vi "Spam - Wait.vi"(8 "Error In":errorcluster, 11 "Spam Frequency":T1=enum."Every 2 ms") -> (0 "Error Out":errorcluster)   [LabVIEW 2016, in "Anti-Spam Tester (AST).lvlib"]
doc: "Blank VI with error handling."
uses:
  Anti-Spam Tester (AST).lvlib
  Spam Frequency (enum).ctl
panel:
  # "Input\nInputs to the VI"
  # "Development\nControls or indicators that are useful for development or testing, but which are not outputs of the VI."
  # "Output\nOutputs of the VI"
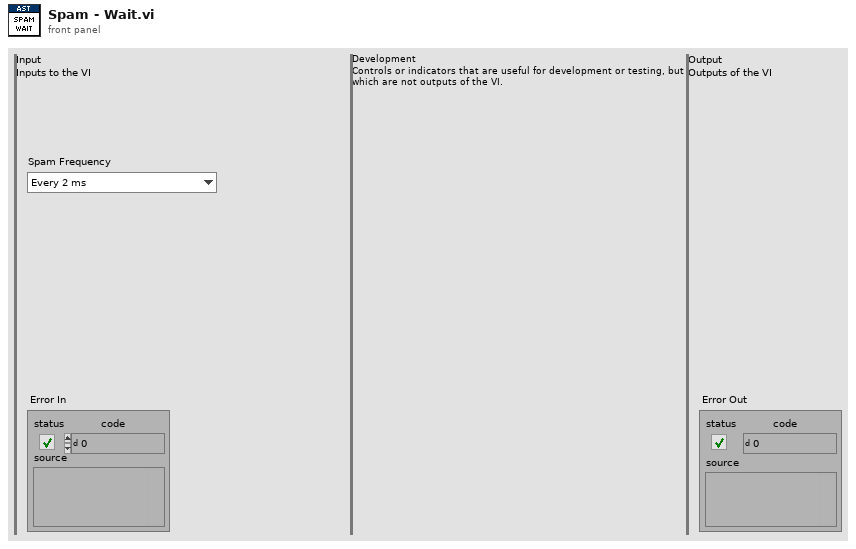
[diagram p1: front panel]
types:
  T1 = typedef "Anti-Spam Tester (AST).lvlib/Spam Frequency (enum).ctl" = enum16{"As fast as possible", "Every 1 ms", "Every 2 ms", "Every 5 ms", "Every 10 ms", "Every 20 ms", "Every 50 ms", "Every 100 ms", "Every 200 ms", "Every 500 ms", "Every 1000 ms"}
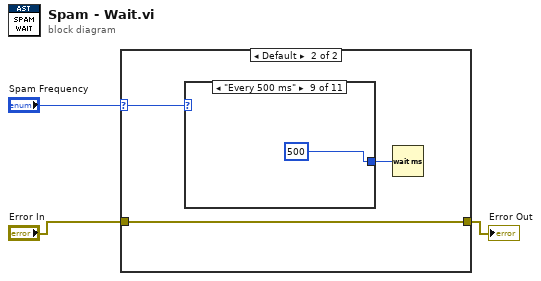
[diagram p0: block diagram]
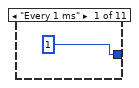
[diagram p3: hidden frame]
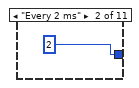
[diagram p4: hidden frame]
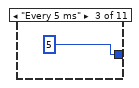
[diagram p5: hidden frame]
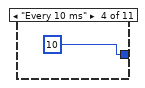
[diagram p6: hidden frame]
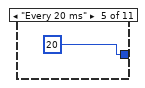
[diagram p7: hidden frame]
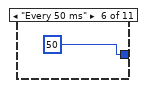
[diagram p8: hidden frame]
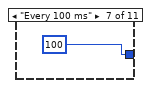
[diagram p9: hidden frame]
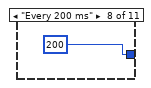
[diagram p10: hidden frame]
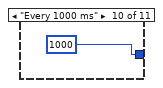
[diagram p11: hidden frame]
diagram:
  n1 = case shown="Default" "Spam Frequency" {
    selector: "Spam Frequency" -> [_ w6]
    tunnel: [w4 w7] -> w2
    tunnel: "Error In" -> [w4 w7]
    frame "As fast as possible" {
    }
    frame Default {
      n2 = case shown="\"Every 500 ms\"" w6 {
        tunnel: [u32 1 ("milliseconds to wait") u32 2 ("milliseconds to wait") u32 5 ("milliseconds to wait") u32 10 ("milliseconds to wait") u32 20 ("milliseconds to wait") u32 50 ("milliseconds to wait") u32 100 ("milliseconds to wait") u32 200 ("milliseconds to wait") u32 500 ("milliseconds to wait") u32 1000 ("milliseconds to wait") _] -> w5
        frame "Every 1 ms" {
        }
        frame "Every 2 ms" {
        }
        frame "Every 5 ms" {
        }
        frame "Every 10 ms" {
        }
        frame "Every 20 ms" {
        }
        frame "Every 50 ms" {
        }
        frame "Every 100 ms" {
        }
        frame "Every 200 ms" {
        }
        frame "Every 500 ms" {
        }
        frame "Every 1000 ms" {
        }
        frame "As fast as possible" {
        }
      }
      n3 = Wait (ms)(milliseconds to wait=w5) -> ()  [unwired: 1 out]
    }
  }
  "Error Out" <- w2
